vi "FaKI State Machine.vi"() -> ()   [LabVIEW 2020, in "Code Cleanup.lvlib" / "FaKI State Machine.lvlib"]
doc: "The Producer-Consumer version of JKI State Machine.\n\nThis VI template must be instantiated by placing it on the block diagram of a new blank VI directly from the palettes. Do not use this template directly."
uses:
  FaKI State Machine.lvlib
panel:
  in  "Exit":bool
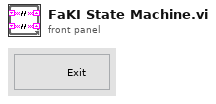
[diagram p1: front panel]
types:
  T1 = enum32{"Invalid", "Standard", "Closed", "Hidden", "Minimized", "Maximized"}
  T2 = enum32{"invalid app kind", "Development System", "Run Time System", "Student Edition", "Embedded LabVIEW", "Evaluation", "Custom"}
  T3 = cluster{"Core":cluster{"Current VI Reference":refnum<vi>, "Close Panel on Exit?":bool}}
  T4 = cluster{"Current VI Reference":refnum<vi>, "Close Panel on Exit?":bool}
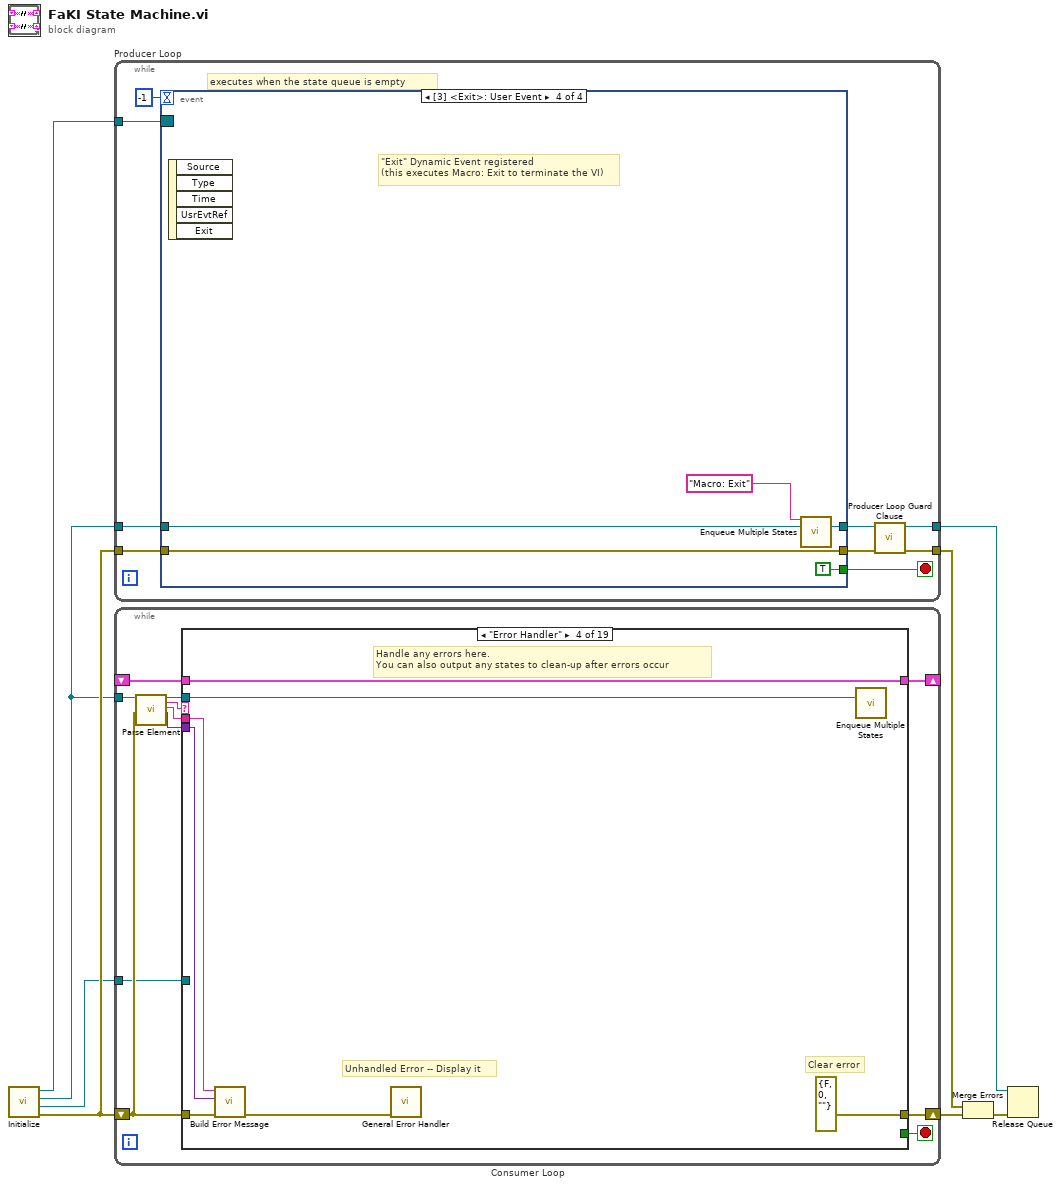
[diagram p0: block diagram]
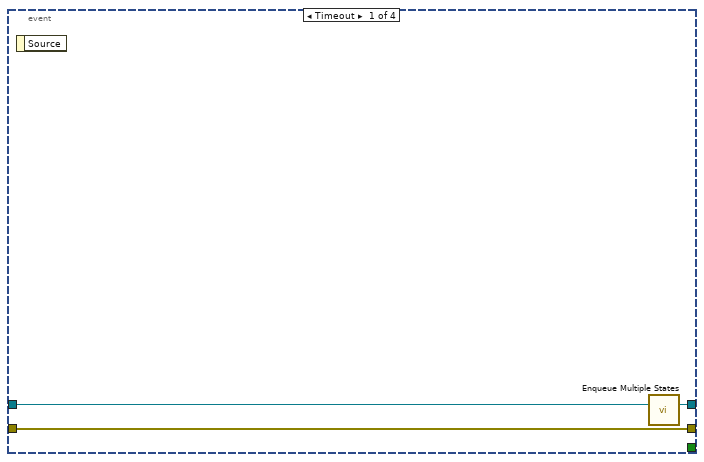
[diagram p2: hidden frame]
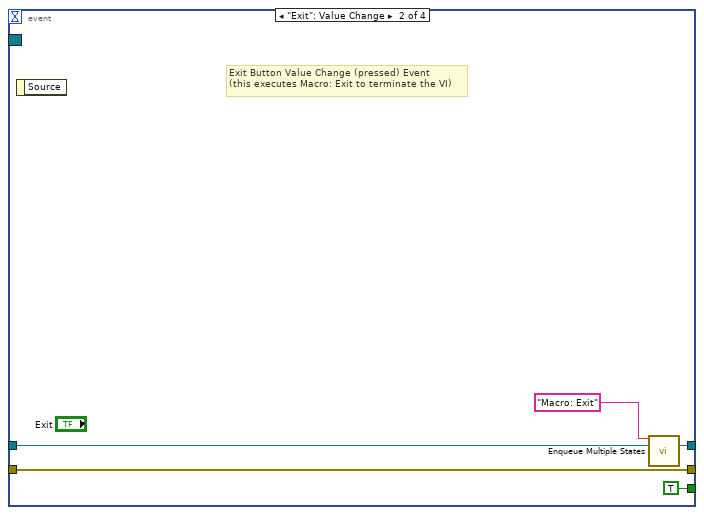
[diagram p3: hidden frame]
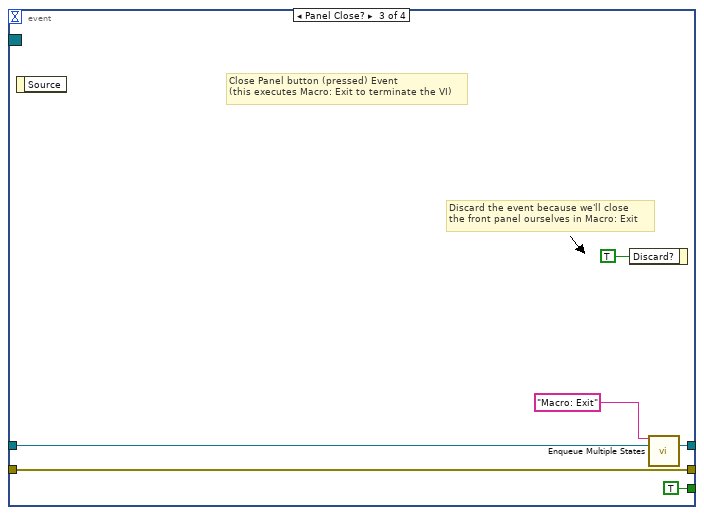
[diagram p4: hidden frame]
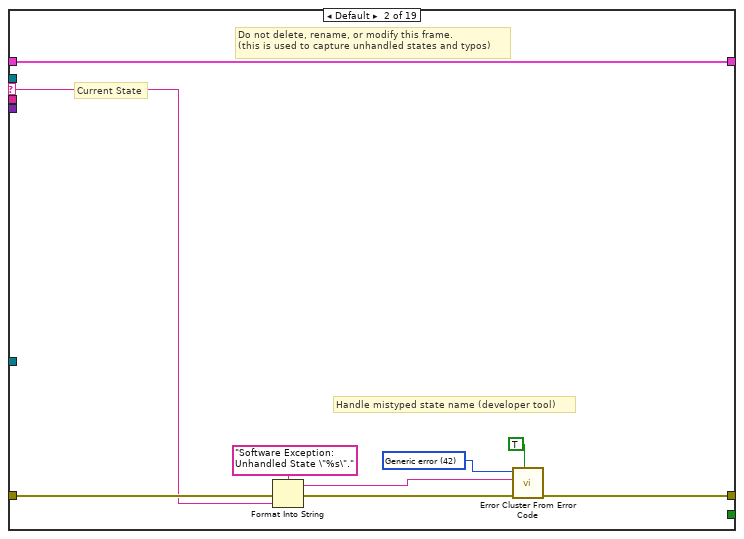
[diagram p6: hidden frame]
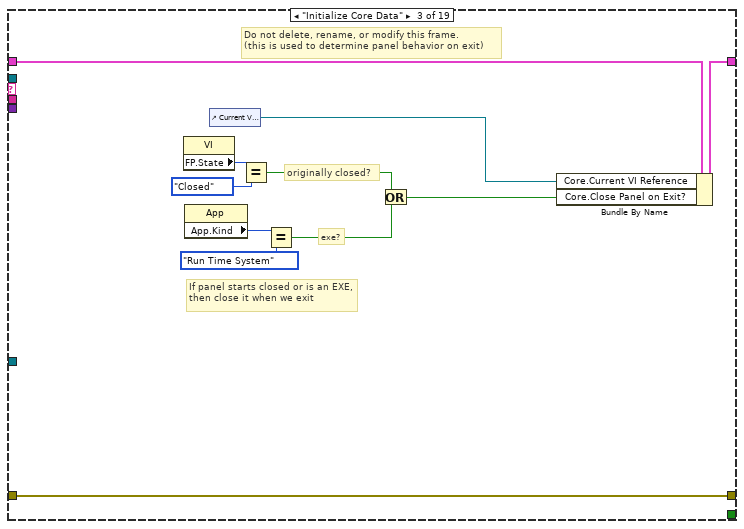
[diagram p7: hidden frame]
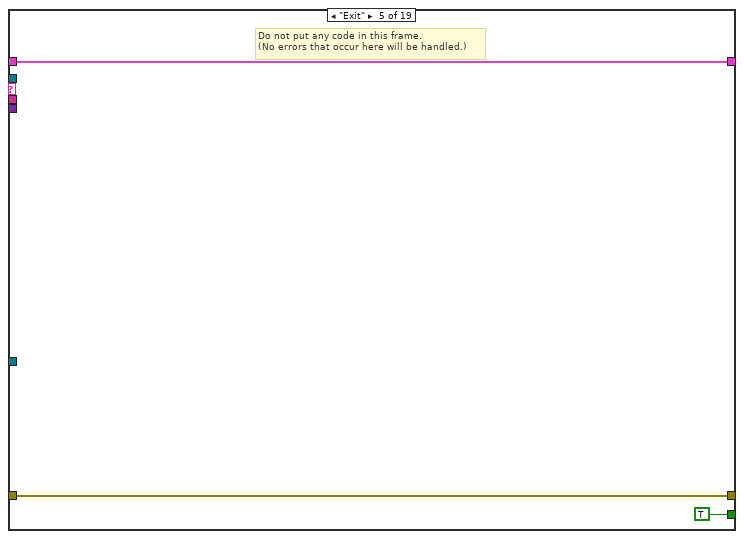
[diagram p8: hidden frame]
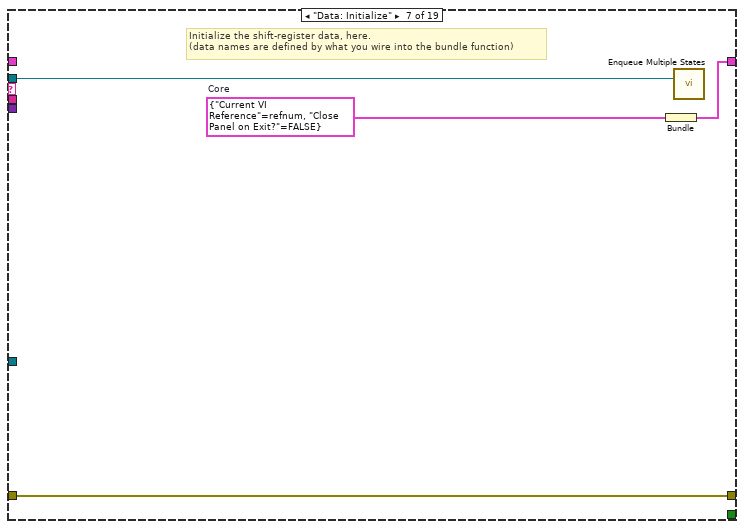
[diagram p10: hidden frame]
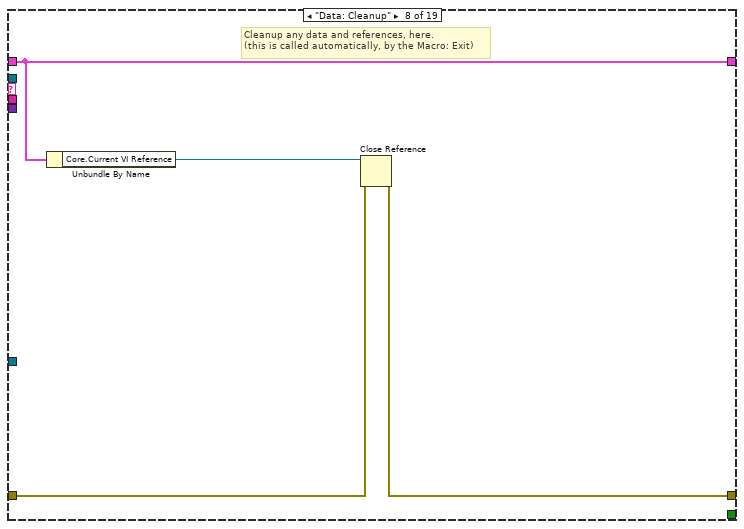
[diagram p11: hidden frame]
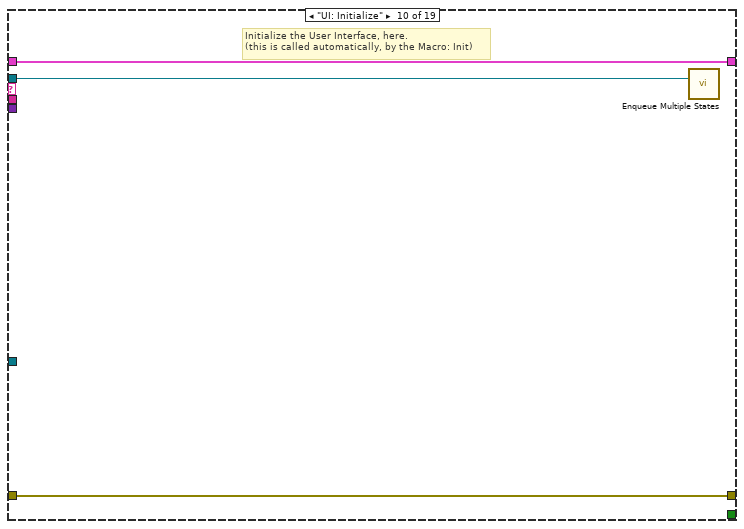
[diagram p13: hidden frame]
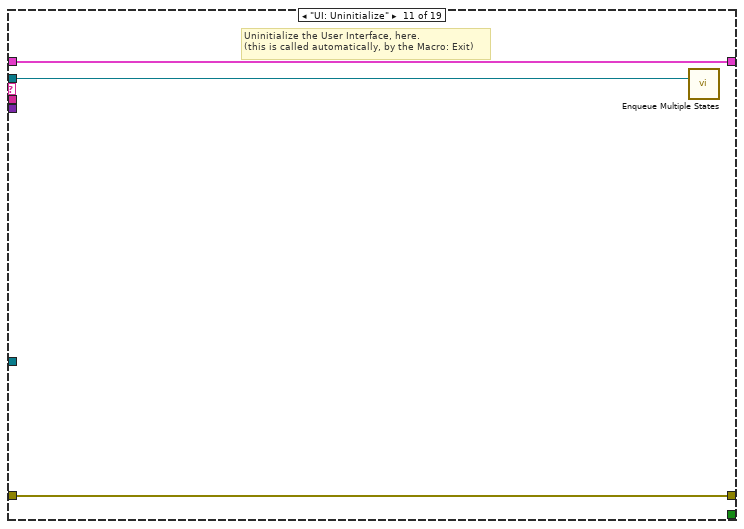
[diagram p14: hidden frame]
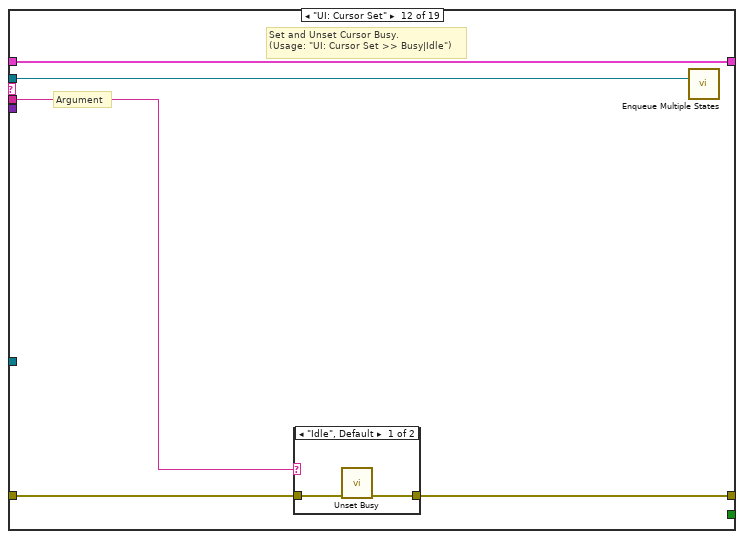
[diagram p15: hidden frame]
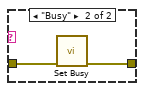
[diagram p16: hidden frame]
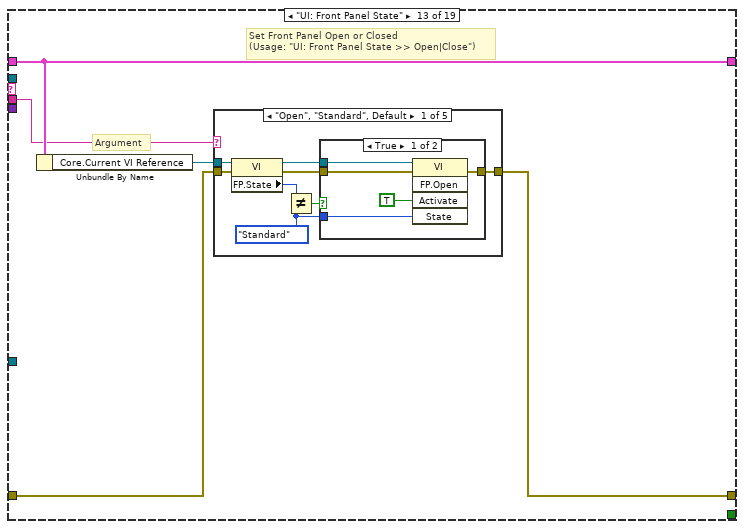
[diagram p17: hidden frame]
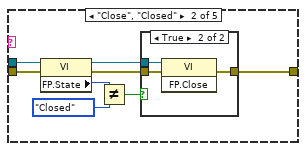
[diagram p19: hidden frame]
diagram:
  n1 = call "Initialize.vi"() -> ("error out"=w4:errorcluster, "Exit Event"=w3:refnum<user-event>, "Queue"=w2:refnum<queue>, "Event Registration Refnum"=w1:refnum<event-registration>)  [unwired: 8 in]
  n2 = while "Producer Loop" {
    tunnel: w1 -> [w9]
    tunnel: w2 -> [w15]
    tunnel: [w10] -> w5
    tunnel: w4 -> [w17]
    tunnel: [w12] -> w7
    stop <- w14 stop-if-true
    # "executes when the state queue is empty"
    n3 = event shown="[3] <Exit>: User Event" {
      selector: w9 -> [_ _ _ _]
      dyn-events: _ -> [_ _ _ _]
      timeout: -1 ("Timeout") -> [_ _ _ _]
      tunnel: [w18 w25 w31 w36] -> w13
      tunnel: w17 -> [w18 w25 w31 w36]
      tunnel: w15 -> [w19 w24 w28 w34]
      tunnel: [w20 w22 w27 w33] -> w11
      tunnel: [_ TRUE TRUE TRUE] -> w14
      event Timeout {
        n4 = event-data() -> ()  [unwired: 1 in, 1 out]
        n5 = call "Enqueue Multiple States.vi"("queue in"=w19) -> ("queue out"=w20:refnum<queue>)  [unwired: 14 in]
      }
      event "Exit": Value Change {
        # "Exit Button Value Change (pressed) Event\n(this executes Macro: Exit to terminate the VI)"
        n6 = event-data() -> ()  [unwired: 1 in, 1 out]
        n7 = call "Enqueue Multiple States.vi"("State(s) at Front"="Macro: Exit", "queue in"=w24) -> ("queue out"=w22:refnum<queue>)  [unwired: 13 in]
      }
      event Panel Close? {
        # "Discard the event because we'll close\nthe front panel ourselves in Macro: Exit"
        # "Close Panel button (pressed) Event\n(this executes Macro: Exit to terminate the VI)"
        n8 = event-data() -> ()  [unwired: 1 in, 1 out]
        n9 = event-data("Discard?"=TRUE) -> ()  [unwired: 1 in, 1 out]
        n10 = call "Enqueue Multiple States.vi"("State(s) at Front"="Macro: Exit", "queue in"=w28) -> ("queue out"=w27:refnum<queue>)  [unwired: 13 in]
      }
      event User Event {
        # "\"Exit\" Dynamic Event registered\n(this executes Macro: Exit to terminate the VI)"
        n11 = event-data() -> ()  [unwired: 1 in, 5 out]
        n12 = call "Enqueue Multiple States.vi"("State(s) at Front"="Macro: Exit", "queue in"=w34) -> ("queue out"=w33:refnum<queue>)  [unwired: 13 in]
      }
    }
    n13 = call "Producer Loop Guard Clause.vi"("error in (no error)"=w13, "queue in"=w11) -> ("error out"=w12:errorcluster, "queue out"=w10:refnum<queue>)  [unwired: 8 in]
  }
  n14 = while "Consumer Loop" {
    shift-right: [w44] -> _
    shift-left: _ -> [w43]
    shift-right: [w47] -> w8
    shift-left: w4 -> [w46]
    tunnel: w2 -> [w42]
    tunnel: w3 -> [w37]
    stop <- w45 stop-if-true
    n15 = call "Parse Element.vi"("queue in"=w42, "error in (no error)"=w46) -> ("queue out"=w41:refnum<queue>, "State"=w40:string, "Arg"=w39:string, "Data"=w38:variant)  [unwired: 14 in]
    n16 = case shown="\"Error Handler\"" w40 {
      selector: w40 -> [_ w50 _ _ _ _ _ _ _ _ _ _ _ _ _ _ _ _ _]
      tunnel: w41 -> [_ _ _ w74 _ _ w82 _ _ w92 w95 w98 _ _ w180 w187 _ w195 w198]
      tunnel: w39 -> [_ _ _ w70 _ _ _ _ _ _ _ w99 w107 _ _ _ _ _ _]
      tunnel: w43 -> [w48 w52 w64 w75 w78 w80 _ w86 w90 w93 w96 w100 w109 w177 w181 w191 w193 w196 w199]
      tunnel: [w49 w57 w69 errorcluster {"status"=FALSE, "code"=0, "source"=""} ("error out") w79 w81 w85 w88 w91 w94 w97 w101 w110 w178 w182 w192 w194 w197 w200] -> w47
      tunnel: w46 -> [w49 w56 w69 w73 w79 w81 w85 w89 w91 w94 w97 w102 w111 w178 w182 w192 w194 w197 w200]
      tunnel: [_ _ _ _ TRUE _ _ _ _ _ _ _ _ _ _ _ _ _ _] -> w45
      tunnel: [w48 w52 w68 w75 w78 w80 w84 w86 w90 w93 w96 w100 w109 w177 w181 w191 w193 w196 w199] -> w44
      tunnel: w38 -> [_ _ _ w71 _ _ _ _ _ _ _ _ _ _ _ _ _ _ _]
      tunnel: w37 -> [_ _ _ _ _ _ _ _ _ _ _ _ _ _ _ _ _ _ _]
      frame "---------- Core ----------" {
        # "Do not put any code in this frame.\n(it is a separator no-op)"
      }
      frame Default {
        w54 = 42 items=["No error", "Argument error", "Memory is full", "Out of zone", "End of file", "File already open", "Generic file I/O error", "File not found", "File permission error", "Disk is full", "Duplicate path", "Too many files open", "System feature not enabled", "Resource file not found", "Cannot add resource", "Resource not found", "Image not found", "Image memory error", "Pen does not exist", "Config type invalid", "Config token not found", "Config parse error", "Config memory error", "Bad external code format", "Bad external code offset", "External code not present", "Null window", "Destroy window error", "Null menu", "Print aborted", "Bad print record", "Print driver error", "Windows error during printing", "Memory error during printing", "Print dialog error", "Generic print error", "Invalid device refnum", "Device not found", "Device parameter error", "Device unit error", "Cannot open device", "Device call aborted", "Generic error", "Cancelled by user", "Object ID too low", "Object ID too high", "Object not in heap", "Unknown heap", "Unknown object (invalid DefProc)", "Unknown object (DefProc not in table)", "Message out of range", "Invalid (null) method", "Unknown message", "Manager call not supported", "Bad address", "Network operation in progress", "Network operation timed out", "Connection is busy", "Network attribute not supported", "Network error", "Address in use", "System out of memory", "Connection aborted", "Connection refused", "Not connected", "Already connected", "Connection closed", "Initialization error (interapplication manager)", "Bad occurrence", "Wait on unbound occurrence handler", "Occurrence queue overflow", "Datalog type conflict", "Unused", "Unrecognized type (interapplication manager)", "Memory corrupt", "Failed to make temporary DLL", "Old CIN version", "Drag socket not found", "Failed to load drop-object", "Failed to register OLE object", "Failed to release OLE object", "Format specifier type mismatch", "Unknown format specifier", "Too few format specifiers", "Too many format specifiers", "Scan failed", "Newer CIN version", "Error converting to variant", "Runtime menu error", "Password tampered", "Variant attribute not found", "Incompatible variant data type", "Event data is not available", "Event Store is not present", "Occurrence is not found", "Event Queue is not created", "Event info is not available", "Refnum passed is NULL", "Error retrieving Class GUID", "Error retrieving CoClass GUID", "Error retrieving TypeLib GUID.", "Bad built application magic bytes.", "Specific driver is different from the specific driver associated with the Logical Name.", "There is no session opened to the class driver.", "Max Error", "MAX - Error with config objects", "MAX - Error loading configuration", "MAX - Group not supported"]
        # "Current State"
        # "Do not delete, rename, or modify this frame.\n(this is used to capture unhandled states and typos)"
        # "Handle mistyped state name (developer tool)"
        n17 = Format Into String(format string="Software Exception: Unhandled State \"%s\"." ("message"), error in=w56, w50) -> (resulting string=w53:string, error out=w58:errorcluster)  [unwired: 1 in]
        n18 = call <vilib>:"Error Cluster From Error Code.vi"("show call chain? (False)"=TRUE, "error in (no error)"=w58, "error message (\"\")"=w53, "error code (0)"=w54) -> ("error out"=w57:errorcluster)  [unwired: 5 in]
      }
      frame "Initialize Core Data" {
        # "Do not delete, rename, or modify this frame.\n(this is used to determine panel behavior on exit)"
        # "originally closed?"
        # "exe?"
        # "If panel starts closed or is an EXE, then close it when we exit"
        n19 = property class="VI"() -> ("FP.State"=w61:T1)  [unwired: 2 in, 2 out]
        n20 = property class="App"() -> ("App.Kind"=w67:T2)  [unwired: 2 in, 2 out]
        n21 = control-ref of="Current VI Reference"() -> (w62:refnum<vi>)
        n22 = Equal?(x=w61, y=T1."Closed" ("Front Panel Window:State")) -> (x = y?=w59:bool)
        n23 = Equal?(x=w67, y=T2."Run Time System" ("Application:Kind")) -> (x = y?=w65:bool)
        n24 = Or(x=w59, y=w65) -> (x .or. y?=w63:bool)
        n25 = Bundle By Name(cluster=w64, "Core.Current VI Reference"=w62, "Core.Close Panel on Exit?"=w63) -> (w68:T3)
      }
      frame "Error Handler" {
        # "Unhandled Error -- Display it"
        # "Handle any errors here.\nYou can also output any states to clean-up after errors occur"
        # "Clear error"
        n26 = call "Build Error Message.vi"("error in (no error)"=w73, "Data"=w71, "Arg"=w70) -> ("error out"=w72:errorcluster)  [unwired: 8 in]
        n27 = call <vilib>:"General Error Handler.vi"("error in (no error)"=w72) -> ()  [unwired: 10 in, 5 out]
        n28 = call "Enqueue Multiple States.vi"("queue in"=w74) -> ()  [unwired: 14 in, 1 out]
      }
      frame "Exit" {
        # "Do not put any code in this frame.\n(No errors that occur here will be handled.)"
      }
      frame "---------- Data ----------" {
        # "Do not put any code in this frame.\n(It is a separator no-op. You can make a copy of this frame to create a new Data frame)"
      }
      frame "Data: Initialize" {
        w83 = T4 {"Current VI Reference"=refnum, "Close Panel on Exit?"=FALSE}  # Core
        # "Initialize the shift-register data, here.\n(data names are defined by what you wire into the bundle function)"
        n29 = Bundle("Core"=w83) -> (w84:T3)  [unwired: 1 in]
        n30 = call "Enqueue Multiple States.vi"("queue in"=w82) -> ()  [unwired: 14 in, 1 out]
      }
      frame "Data: Cleanup" {
        # "Cleanup any data and references, here.\n(this is called automatically, by the Macro: Exit)"
        n31 = Unbundle By Name(w86) -> ("Core.Current VI Reference"=w87:refnum<vi>)
        n32 = Close Reference(reference=w87, error in (no error)=w89) -> (error out=w88:errorcluster)
      }
      frame "---------- UI ----------" {
        # "Do not put any code in this frame.\n(It is a separator no-op. You can make a copy of this frame to create a new UI frame)"
      }
      frame "UI: Initialize" {
        # "Initialize the User Interface, here.\n(this is called automatically, by the Macro: Init)"
        n33 = call "Enqueue Multiple States.vi"("queue in"=w92) -> ()  [unwired: 14 in, 1 out]
      }
      frame "UI: Uninitialize" {
        # "Uninitialize the User Interface, here.\n(this is called automatically, by the Macro: Exit)"
        n34 = call "Enqueue Multiple States.vi"("queue in"=w95) -> ()  [unwired: 14 in, 1 out]
      }
      frame "UI: Cursor Set" {
        # "Argument"
        # "Set and Unset Cursor Busy.\n(Usage: \"UI: Cursor Set >> Busy|Idle\")"
        n35 = case shown="\"Idle\", Default" w99 {
          tunnel: w102 -> [w104 w106]
          tunnel: [w103 w105] -> w101
          frame "Idle", Default {
            n36 = call <vilib>:"Unset Busy.vi"("error in (no error)"=w104) -> ("error out"=w103:errorcluster)  [unwired: 10 in]
          }
          frame "Busy" {
            n37 = call <vilib>:"Set Busy.vi"("error in (no error)"=w106) -> ("error out"=w105:errorcluster)  [unwired: 9 in, 1 out]
          }
        }
        n38 = call "Enqueue Multiple States.vi"("queue in"=w98) -> ()  [unwired: 14 in, 1 out]
      }
      frame "UI: Front Panel State" {
        # "Argument"
        # "Set Front Panel Open or Closed\n(Usage: \"UI: Front Panel State >> Open|Close\")"
        n39 = Unbundle By Name(w109) -> ("Core.Current VI Reference"=w108:refnum<vi>)
        n40 = case shown="\"Open\", \"Standard\", Default" w107 {
          tunnel: w111 -> [w118 w132 w144 w157 w170]
          tunnel: [w119 w133 w145 w158 w171] -> w110
          tunnel: w108 -> [w116 w130 w142 w155 w168]
          frame "Open", "Standard", Default {
            w112 = T1."Standard" ("State")
            n41 = property class="VI"(reference=w116, error in=w118) -> (reference out=w115:refnum<vi>, error out=w117:errorcluster, "FP.State"=w114:T1)
            n42 = Not Equal?(x=w114, y=w112) -> (x != y?=w113:bool)
            n43 = case shown="True" w113 {
              tunnel: [w124 w125] -> w119
              tunnel: w117 -> [w123 w125]
              tunnel: w115 -> [w121 _]
              tunnel: w112 -> [w120 _]
              frame True {
                n44 = invoke class="VI" method="FP.Open"(reference=w121, error in=w123, "Activate"=TRUE, "State"=w120) -> (error out=w124:errorcluster)  [unwired: 1 in, 4 out]
              }
              frame False {
              }
            }
          }
          frame "Close", "Closed" {
            n45 = property class="VI"(reference=w130, error in=w132) -> (reference out=w129:refnum<vi>, error out=w131:errorcluster, "FP.State"=w127:T1)
            n46 = Not Equal?(x=w127, y=T1."Closed" ("Front Panel Window:State")) -> (x != y?=w126:bool)
            n47 = case shown="True" w126 {
              tunnel: [w134 w137] -> w133
              tunnel: w131 -> [w134 w136]
              tunnel: w129 -> [_ w135]
              frame False {
              }
              frame True {
                n48 = invoke class="VI" method="FP.Close"(reference=w135, error in=w136) -> (error out=w137:errorcluster)  [unwired: 1 in, 2 out]
              }
            }
          }
          frame "Hidden", "Hide" {
            w138 = T1."Hidden" ("State")
            n49 = property class="VI"(reference=w142, error in=w144) -> (reference out=w141:refnum<vi>, error out=w143:errorcluster, "FP.State"=w140:T1)
            n50 = Not Equal?(x=w140, y=w138) -> (x != y?=w139:bool)
            n51 = case shown="True" w139 {
              tunnel: [w149 w150] -> w145
              tunnel: w143 -> [w148 w150]
              tunnel: w141 -> [w147 _]
              tunnel: w138 -> [w146 _]
              frame True {
                n52 = invoke class="VI" method="FP.Open"(reference=w147, error in=w148, "State"=w146) -> (error out=w149:errorcluster)  [unwired: 2 in, 4 out]
              }
              frame False {
              }
            }
          }
          frame "Minimize", "Minimized" {
            w151 = T1."Minimized" ("State")
            n53 = property class="VI"(reference=w155, error in=w157) -> (reference out=w154:refnum<vi>, error out=w156:errorcluster, "FP.State"=w153:T1)
            n54 = Not Equal?(x=w153, y=w151) -> (x != y?=w152:bool)
            n55 = case shown="True" w152 {
              tunnel: [w162 w163] -> w158
              tunnel: w156 -> [w161 w163]
              tunnel: w154 -> [w160 _]
              tunnel: w151 -> [w159 _]
              frame True {
                n56 = invoke class="VI" method="FP.Open"(reference=w160, error in=w161, "State"=w159) -> (error out=w162:errorcluster)  [unwired: 2 in, 4 out]
              }
              frame False {
              }
            }
          }
          frame "Maximize", "Maximized" {
            w164 = T1."Maximized" ("State")
            n57 = property class="VI"(reference=w168, error in=w170) -> (reference out=w167:refnum<vi>, error out=w169:errorcluster, "FP.State"=w166:T1)
            n58 = Not Equal?(x=w166, y=w164) -> (x != y?=w165:bool)
            n59 = case shown="True" w165 {
              tunnel: [w175 w176] -> w171
              tunnel: w169 -> [w174 w176]
              tunnel: w167 -> [w173 _]
              tunnel: w164 -> [w172 _]
              frame True {
                n60 = invoke class="VI" method="FP.Open"(reference=w173, error in=w174, "State"=w172) -> (error out=w175:errorcluster)  [unwired: 2 in, 4 out]
              }
              frame False {
              }
            }
          }
        }
      }
      frame "---------- Macro ----------" {
        # "Do not put any code in this frame.\n(It is a separator no-op. You can make a copy of this frame to create a new Macro frame)"
      }
      frame "Macro: Initialize" {
        w179 = "Data: Initialize\nInitialize Core Data\nUI: Initialize\nUI: Front Panel State >> Open"  # Data: Initialize Initialize Core Data UI: Initialize UI: Front Panel State >> Open
        # "Initialization Macro\n(This is called once, when the VI starts)"
        n61 = call "Enqueue Multiple States.vi"("State(s) at Front"=w179, "queue in"=w180) -> ()  [unwired: 13 in, 1 out]
      }
      frame "Macro: Exit" {
        # "Exit Macro\n(This is called once, when the VI exits)"
        n62 = Unbundle By Name(w191) -> ("Core.Close Panel on Exit?"=w190:bool)
        n63 = Select(t="UI: Front Panel State >> Close\n", s=w190, f="") -> (s? t:f=w186:string)
        n64 = Concatenate Strings("UI: Uninitialize\n", w186, "Data: Cleanup\nExit") -> (w184:string)
        n65 = call "Enqueue Multiple States.vi"("State(s) at Front"=w184, "queue in"=w187) -> ()  [unwired: 13 in, 1 out]
      }
      frame "---------- New Category ----------" {
        # "Template Separator\n(You can make a copy of, or modify, this frame)"
      }
      frame "New Category: 1" {
        # "Your code here.\n(You can make a copy of, or modify, this frame)"
        n66 = call "Enqueue Multiple States.vi"("queue in"=w195) -> ()  [unwired: 14 in, 1 out]
      }
      frame "New Category: 2" {
        # "Your code here.\n(You can make a copy of, or modify, this frame)"
        n67 = call "Enqueue Multiple States.vi"("queue in"=w198) -> ()  [unwired: 14 in, 1 out]
      }
    }
  }
  n68 = Merge Errors(w7, w8) -> (w6:errorcluster)
  n69 = Release Queue(queue=w5, error in (no error)=w6) -> ()  [unwired: 1 in, 3 out]
